vi "Get Resource Purpose.vi"(11 "Resource in":refnum<class "Resource.lvclass">) -> (2 "Resource Purpose":string)   [LabVIEW 2020, in "CTI.lvlib" / "Resource.lvclass"]
uses:
  Resource.lvclass
  Resource.lvclass/Resource.ctl
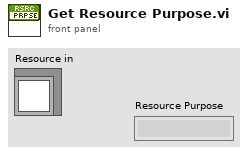
[diagram p1: front panel]
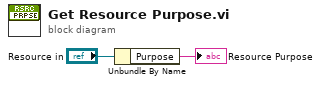
[diagram p0: block diagram]
diagram:
  n1 = Unbundle By Name("Resource in") -> ("Purpose"=→"Resource Purpose":string)
